vi "Query Voltage Copy.vi"(8 "error in (no error)":errorcluster, 10 "Channel (0: Channel 1)":T1 items=["Channel 1", "Channel 2"], 11 "VISA resource name":refnum<visa-resource-name>) -> (0 "error out":errorcluster, 1 "voltage copy?":bool, 3 "VISA resource name out":refnum<visa-resource-name>)   [LabVIEW 2009, in "Tektronix AFG 3000 Series.lvlib"]
doc: "Queries whether voltage copying is turned on or off. This feature allows you to copy the voltage level of one channel to another channel. The channel specified in the command is copied to the other channel, and the other channel's voltage levels mirror the original until copying is turned off."
uses:
  Tektronix AFG 3000 Series.lvlib
  controls.llb/Channel.ctl
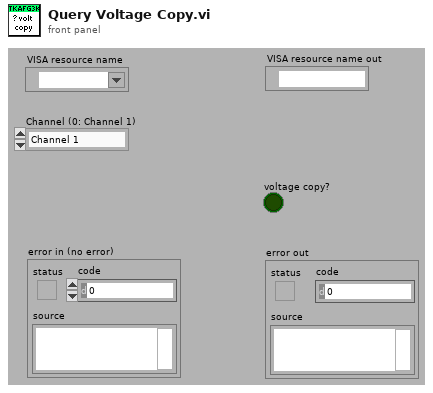
[diagram p1: front panel]
types:
  T1 = typedef "Channel.ctl" = u16
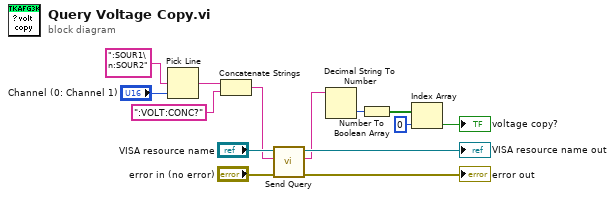
[diagram p0: block diagram]
diagram:
  n1 = Pick Line(multi-line string=":SOUR1\n:SOUR2", line index="Channel (0: Channel 1)") -> (output string=w11:string)  [unwired: 1 out]
  n2 = Concatenate Strings(w11, ":VOLT:CONC?" ("format string")) -> (w10:string)
  n3 = call "Send Query.vi"("error in (no error)"="error in (no error)", "write buffer"=w10, "VISA resource name"="VISA resource name") -> ("error out"=→"error out":errorcluster, "read buffer"=w5:string, "VISA resource name out"=→"VISA resource name out":refnum<visa-resource-name>)  [unwired: 1 in, 5 out]
  n4 = Decimal String To Number(string=w5) -> (number=w1:i32)  [unwired: 3 out]
  n5 = Number To Boolean Array(number=w1) -> (Boolean array=w4:bool[])
  n6 = Index Array(array=w4, index=0) -> (element=→"voltage copy?":bool)
